vi "formatIntoRowInterface.vi"(8 "error in (no error)":errorcluster, 11 "Transaction in":refnum<class "Transaction.lvclass">) -> (0 "error out":errorcluster, 3 "Table Row":string[](array[string]))   [LabVIEW 2018, in "Transaction.lvclass"]
uses:
  Transaction.lvclass
  Transaction.lvclass/Transaction.ctl
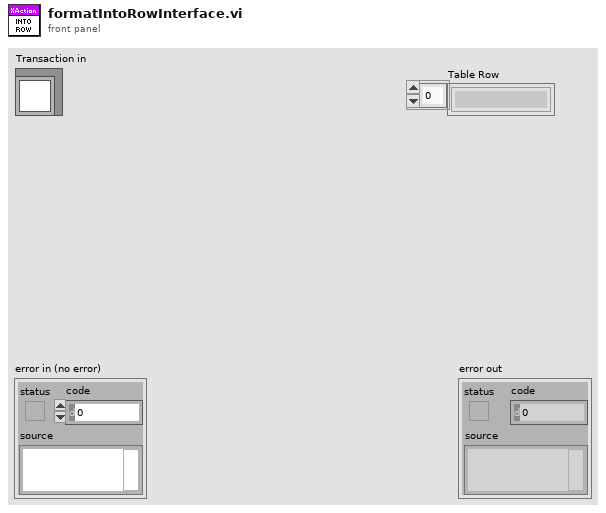
[diagram p1: front panel]
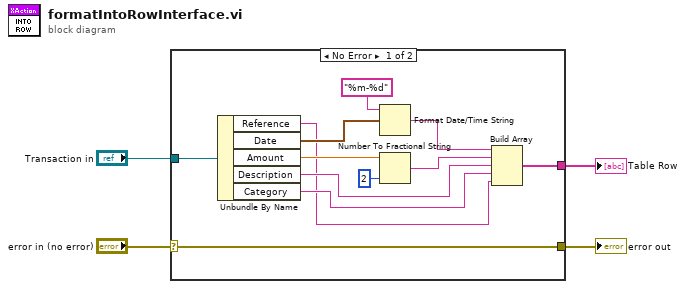
[diagram p0: block diagram]
diagram:
  n1 = case shown="No Error" "error in (no error)" {
    selector: "error in (no error)" -> [w16 w17]
    tunnel: [w16 w17] -> w3
    tunnel: "Transaction in" -> [w15 _]
    tunnel: [w10 _] -> w1
    frame No Error {
      n2 = Unbundle By Name(w15) -> ("Reference"=w5:string, "Date"=w14:timestamp, "Amount"=w9:dbl, "Description"=w7:string, "Category"=w6:string)
      n3 = Format Date/Time String(time format string (%c)="%m-%d", seconds (now)=w14) -> (date/time string=w11:string)  [unwired: 1 in]
      n4 = Number To Fractional String(number=w9, precision (6)=i16 2) -> (F-format string=w8:string)  [unwired: 2 in]
      n5 = Build Array(w11, w8, w7, w6, w5) -> (w10:string[])
    }
    frame Error {
    }
  }
  "error out" <- w3
  "Table Row" <- w1
